vi "DeCoF string query.vi"(4 "error in":errorcluster, 5 "use gsv":bool, 6 "param-name":string, 7 "Conncection ID in":T1) -> (0 "error out":errorcluster, 2 "value":string, 3 "Conncection ID out":T1)   [LabVIEW 2013]
uses:
  subVIs/DeCoF connection.ctl
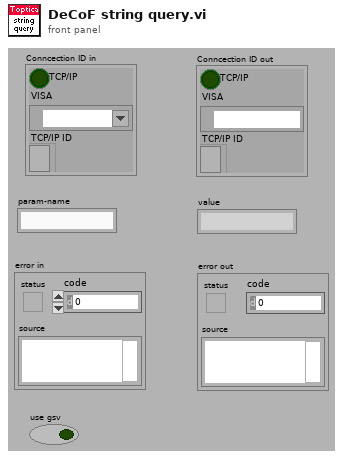
[diagram p1: front panel]
types:
  T1 = typedef "DeCoF connection.ctl" = cluster{"TCP/IP":bool, "VISA":refnum<visa-resource-name>, "TCP/IP ID":refnum<k5>}
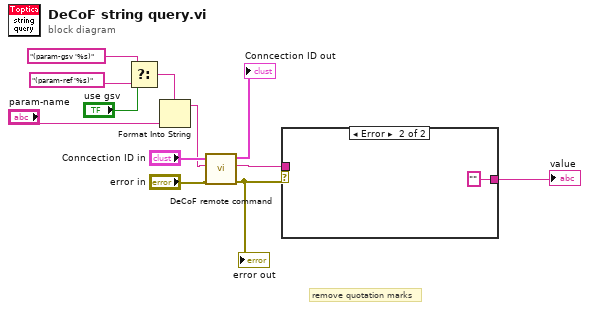
[diagram p0: block diagram]
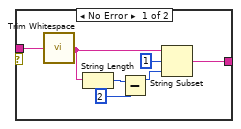
[diagram p2: hidden frame]
diagram:
  # "remove quotation marks"
  n1 = Select(t="(param-gsv '%s)" ("format string"), s="use gsv", f="(param-ref '%s)" ("format string")) -> (s? t:f=w7:string)
  n2 = Format Into String(format string=w7, "param-name") -> (resulting string=w4:string)  [unwired: 2 in, 1 out]
  n3 = call "DeCoF remote command.vi"("error in (no error)"="error in", "command"=w4, "Conncection ID in"="Conncection ID in") -> ("error out"=w1:errorcluster, "answer string"=w3:string, "Conncection ID out"=→"Conncection ID out":T1)  [unwired: 2 in, 2 out]
  "error out" <- w1
  n4 = case shown="Error" w1 {
    tunnel: w3 -> [w14 _]
    tunnel: [w13 "" ("trimmed string")] -> w2
    frame No Error {
      n5 = call <vilib>:"Trim Whitespace.vi"("string"=w14) -> ("trimmed string"=w17:string)  [unwired: 1 in]
      n6 = String Length(string=w17) -> (length=w15:i32)
      n7 = Subtract(x=w15, y=2) -> (x-y=w18:i32)
      n8 = String Subset(string=w17, offset (0)=1, length (rest)=w18) -> (substring=w13:string)
    }
    frame Error {
    }
  }
  "value" <- w2
